vi "Wait Frame Ok.vi"(8 "entrée d'erreur (pas d'erreur)":errorcluster, 11 "Wait_Frame_ERP1 en entrée":refnum<class "Wait_Frame_ERP1.lvclass">) -> (0 "sortie d'erreur":errorcluster, 3 "Wait_Frame_ERP1 en sortie":refnum<class "Wait_Frame_ERP1.lvclass">)   [LabVIEW 2020, in "Library Test.lvlib" / "Wait_Frame_ERP1.lvclass"]
uses:
  Wait_Frame_ERP1.lvclass
  C:/Users/ngarcin/OneDrive - Altyor/Standard TB/Class/Test/Test (Default)/Test (Default).lvclass
  JSON API/JSON Value/Set from JSON string.vi
  Instrument/Instrument (Default)/Class Instrument (Default).lvclass
  JSON API/JSON Value/JSON Value.lvclass
  Wait_Frame_ERP1.lvclass/Wait_Frame_ERP1.ctl
  JSON API/Variant JSON/Variant JSON.lvlib
  JSON API/Get Polymorphic/JSON GetSet.lvlib
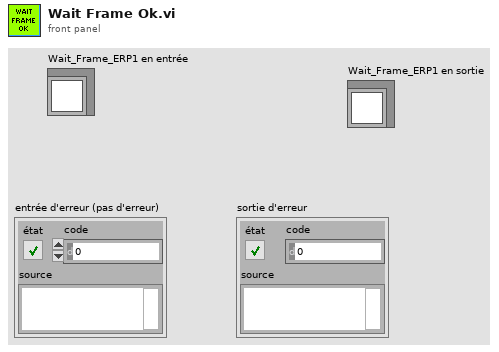
[diagram p1: front panel]
types:
  T1 = cluster{"Frame Read":string, "Frame received":bool, "Frame NOk":bool}
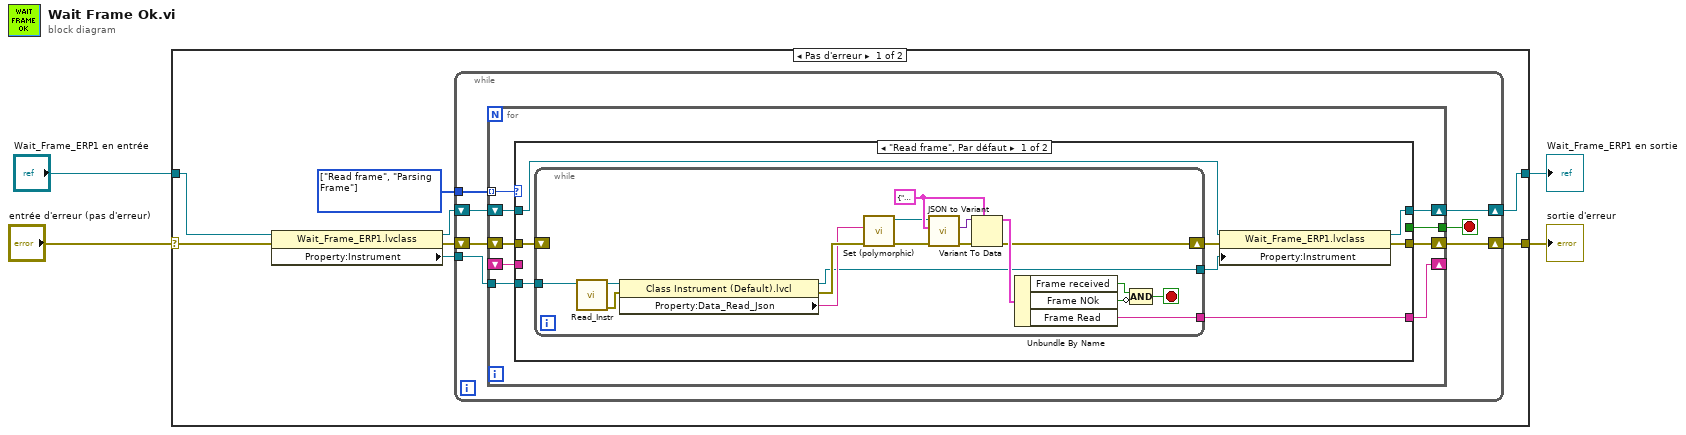
[diagram p0: block diagram]
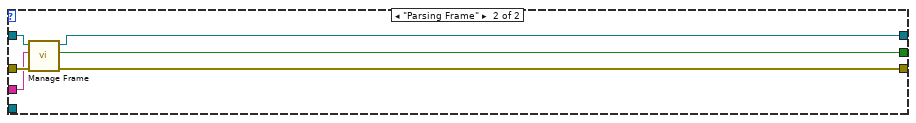
[diagram p2: hidden frame]
diagram:
  n1 = case shown="Pas d'erreur" "entrée d'erreur (pas d'erreur)" {
    selector: "entrée d'erreur (pas d'erreur)" -> [w5 w60]
    tunnel: "Wait_Frame_ERP1 en entrée" -> [w11 w61]
    tunnel: [w7 w60] -> w3
    tunnel: [w6 w61] -> w2
    frame No Error {
      w12 = enum16{"Read frame", "Parsing Frame"}[] [enum."Read frame", enum."Parsing Frame"] items=["Read frame", "Parsing Frame"]
      n2 = property class="Wait_Frame_ERP1.lvclass"(reference=w11, error in=w5) -> (reference out=w8:refnum<class "Wait_Frame_ERP1.lvclass">, error out=w9:errorcluster, "Property:Instrument"=w10:refnum<class "Class Instrument (Default).lvclass">)
      n3 = while {
        tunnel: w12 -> [w19]
        tunnel: w10 -> [w18]
        shift-right: [w15] -> w7
        shift-left: w9 -> [w17]
        shift-right: [w14] -> w6
        shift-left: w8 -> [w16]
        stop <- w13 stop-if-true
        n4 = for {
          tunnel: w18 -> [w27]
          shift-right: [w25] -> w15
          shift-left: w17 -> [w28]
          tunnel: w19 -> [w26] mode=indexing
          shift-right: [w24] -> _
          shift-left: _ -> [w23]
          shift-right: [w21] -> w14
          shift-left: w16 -> [w22]
          tunnel: [w20] -> w13
          n5 = case shown="\"Read frame\", Par défaut" w26 {
            tunnel: [w29 w58] -> w25
            tunnel: [w36 _] -> w24
            tunnel: w28 -> [w35 w59]
            tunnel: w27 -> [w34 _]
            tunnel: w23 -> [_ w57]
            tunnel: w22 -> [w31 w56]
            tunnel: [w30 w55] -> w21
            tunnel: [_ w54] -> w20
            frame "Read frame", Default {
              n6 = while {
                tunnel: [w37] -> w36
                tunnel: w34 -> [w43]
                shift-right: [w38] -> w33
                shift-left: w35 -> [_]
                tunnel: [w39] -> w32
                stop <- w40 stop-if-true
                w52 = T1 {"Frame Read"="", "Frame received"=FALSE, "Frame NOk"=FALSE}
                n7 = call-dynamic "Read_Instr.vi"("Class Instrument (Default) en entrée"=w43) -> ("error out"=w45:errorcluster, "Class Instrument (Default) en sortie"=w44:refnum<class "Class Instrument (Default).lvclass">)  [unwired: 9 in]
                n8 = property class="Class Instrument (Default).lvcl"(reference=w44, error in=w45) -> (reference out=w39:refnum<class "Class Instrument (Default).lvclass">, error out=w50:errorcluster, "Property:Data_Read_Json"=w49:string)
                n9 = call-poly "Set (polymorphic).vi"("error in (no error)"=w50, "JSON stream"=w49) -> ("error out"=w46:errorcluster, "JSON Value out"=w48:refnum<class "JSON Value.lvclass">)  [unwired: 7 in, 1 out]
                n10 = call "JSON to Variant.vi"("error in (no error)"=w46, "Variant (Data Type)"=w52, "JSON Value"=w48) -> ("error out"=w47:errorcluster, "Variant out"=w51:variant)  [unwired: 7 in]
                n11 = Variant To Data(error in=w47, type=w52, Variant=w51) -> (data=w53:T1, error out=w38:errorcluster)
                n12 = Unbundle By Name(w53) -> ("Frame received"=w41:bool, "Frame NOk"=w42:bool, "Frame Read"=w37:string)
                n13 = Compound Arithmetic op=AND ("Opérateur arithmétique")(w41, invert w42) -> (w40:bool)
              }
              n14 = property class="Wait_Frame_ERP1.lvclass"(reference=w31, error in=w33, "Property:Instrument"=w32) -> (reference out=w30:refnum<class "Wait_Frame_ERP1.lvclass">, error out=w29:errorcluster)
            }
            frame "Parsing Frame" {
              n15 = call-dynamic "Manage Frame.vi"("entrée d'erreur (pas d'erreur)"=w59, "Frame Read"=w57, "Wait_Frame_ERP1 en entrée"=w56) -> ("sortie d'erreur"=w58:errorcluster, "Frame Ok"=w54:bool, "Wait_Frame_ERP1 en sortie"=w55:refnum<class "Wait_Frame_ERP1.lvclass">)  [unwired: 6 in]
            }
          }
        }
      }
    }
    frame Error {
    }
  }
  "sortie d'erreur" <- w3
  "Wait_Frame_ERP1 en sortie" <- w2
